vi "Arm Main copy.vi"() -> ()   [LabVIEW 2013]
doc: "This example shows how to move a motor connected to an encoder and a wheel, and then read information about the system from an encoder.\n\nThis is an example of how to use feedback (from the encoder) to create an open loop system. If some control method was used, for example using PID, a closed loop system could be created."
uses:
  Robot Global Data.vi
  Controller 2.vi
panel:
  in  "Movement Incr. Travel":dbl=1.0
  in  "Upper Limit":dbl=0.3 format="%#_13g"
  in  "Lower Limit":dbl=-0.5 format="%#_13g"
  in  "Movement Incr. Picking Up":dbl=1.0
  out "Arm Angle":dbl(graph)=148.31089863414002
  in  "Pickup Position":dbl=90.0
  out "Motor Output":dbl(graph)=0.11689101365859983
  in  "Arm Gain":dbl=0.02
  in  "Multiplier":dbl=1.0
  out "Desired Angle":dbl=160.0
  in  "Travel Position":dbl=160.0
  out "Arm Angle (deg)":dbl(knob)=148.31089863414002 scale=0.0..360.0 scale format="%#_3g"
  # "Output information."
  # "20 msec is drive\nsttion time"
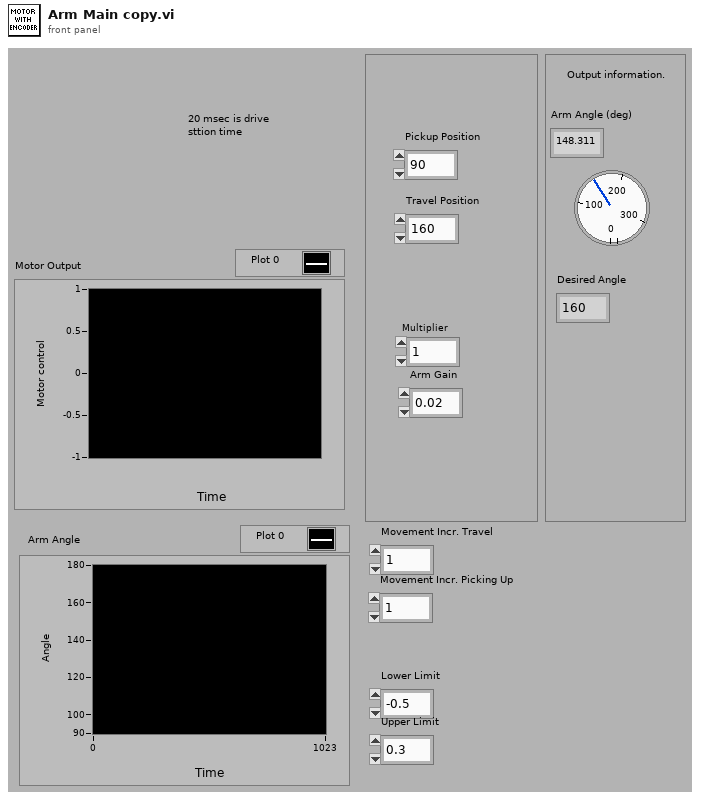
[diagram p1: front panel]
types:
  T1 = cluster{"LS X":dbl, "LS Y":dbl, "Triggers":dbl, "RS X":dbl, "RS Y":dbl}
  T2 = cluster{"A":bool, "B":bool, "X":bool, "Y":bool, "LB":bool, "RB":bool, "Back":bool, "Start":bool, "LS":bool, "RS":bool}
  T3 = typedef "WPI_EncoderDevRef.ctl" = cluster{"DevStatus":errorcluster, "EncoderIndex":T4, "CounterIndex":T5, "DistancePerCount":dbl, "Decoding Type":T6}
  T4 = typedef "FPGA_EncoderIdx.ctl" = enum8{"Enc 0", "Enc 1", "Enc 2", "Enc 3", "Invalid"}
  T5 = typedef "FPGA_CounterCtrSystemIndex.ctl" = enum8{"Ctr 0", "Ctr 1", "Ctr 2", "Ctr 3", "Ctr 4", "Ctr 5", "Ctr 6", "Ctr 7", "Invalid"}
  T6 = typedef "WPI_EncoderType.ctl" = enum16{"1x", "2x", "4x"}
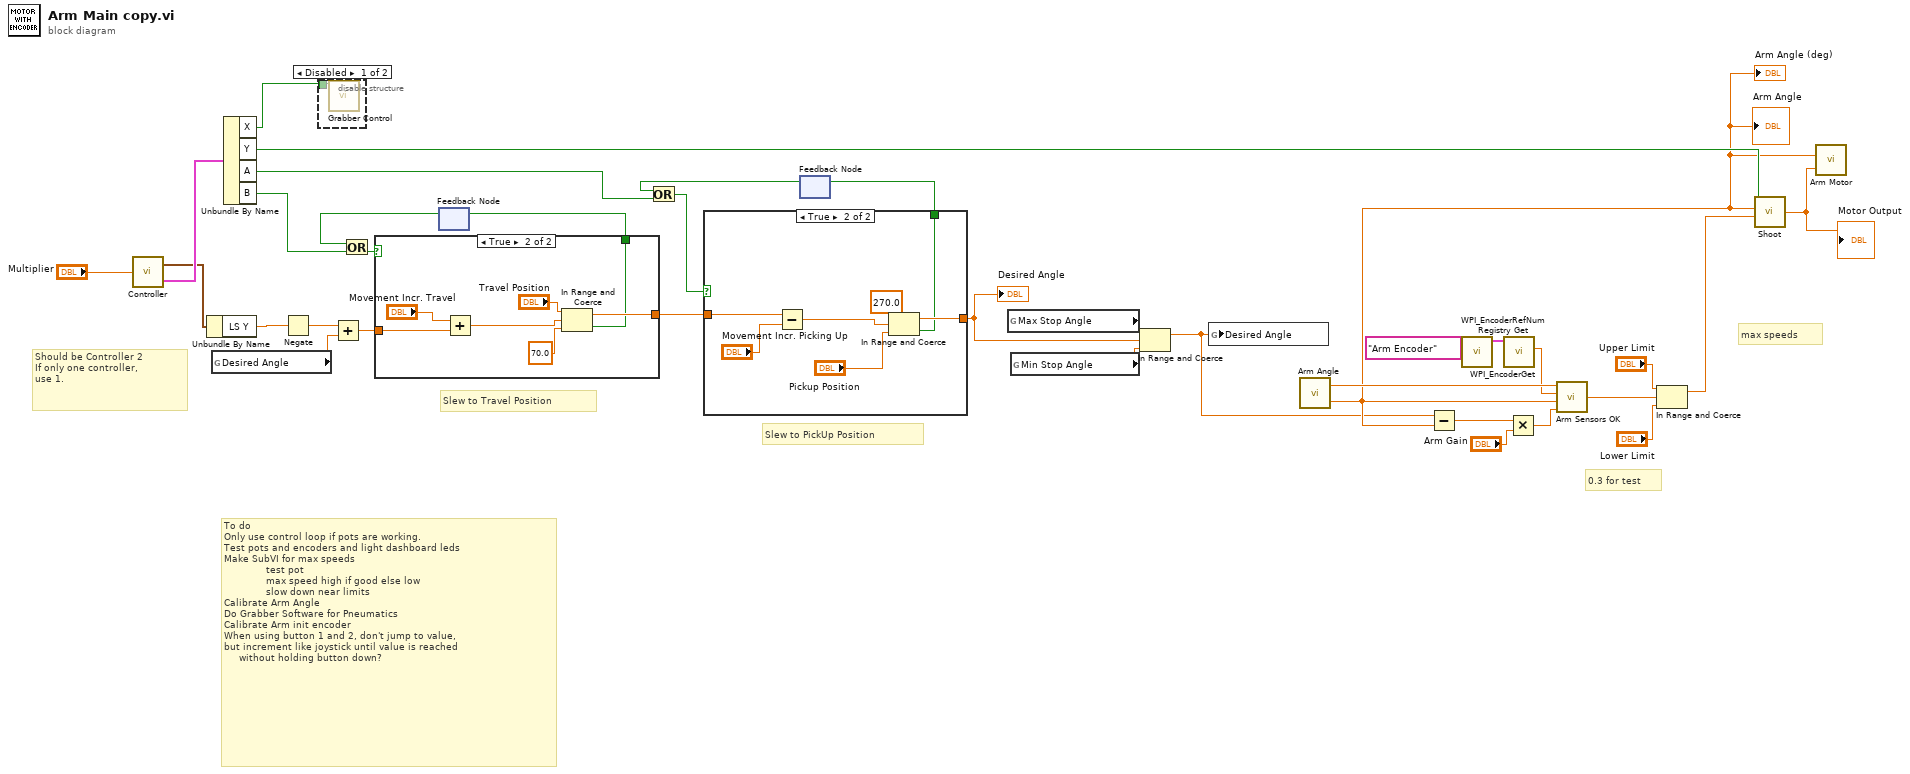
[diagram p0: block diagram]
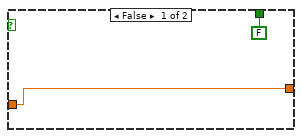
[diagram p3: hidden frame]
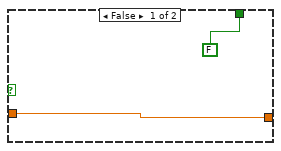
[diagram p4: hidden frame]
diagram:
  # "Slew to PickUp Position"
  # "Slew to Travel Position"
  # "Should be Controller 2\nIf only one controller, \nuse 1."
  # "0.3 for test"
  # "max speeds"
  # "To do\nOnly use control loop if pots are working. \nTest pots and encoders and light dashboard leds\nMake SubVI for max speeds \n              test pot\n              max speed high if good else low\n              slow down near limits\nCalibrate Arm Angle\nDo Grabber Software for Pneumatics\nCalibrate Arm init encoder\nWhen using button 1 and 2, don't jump to value,                                      but increment like joystick until value is reached\n     without holding button down?"
  n1 = call-poly "Controller.vi"("Joystick Multiplier"="Multiplier") -> ("Axes"=w18:T1, "Buttons"=w19:T2)
  n2 = Unbundle By Name(w18) -> ("LS Y"=w16:dbl)
  n3 = global read "Robot Global Data.vi" "Desired Angle"() -> (w9:dbl)
  n4 = Unbundle By Name(w19) -> ("X"=w14:bool, "Y"=w13:bool, "A"=w3:bool, "B"=w15:bool)
  n5 = Negate(x=w16) -> (-x=w32:dbl)
  n6 = disable-structure shown="Disabled" {
    disable-tunnel: w14 -> [w36 _]
    frame Disabled {
      n7 = call "Grabber Control.vi"("Open"=w36) -> ()  [unwired: 2 in]
    }
    frame Enabled {
    }
  }
  n8 = Add(x=w32, y=w9) -> (x+y=w28:dbl)
  n9 = feedback #1() -> (w5:bool)  [unwired: 1 in]
  n10 = Or(x=w5, y=w15) -> (x .or. y?=w7:bool)
  n11 = case shown="True" w7 {
    tunnel: [w38 w42] -> w27
    tunnel: w28 -> [w38 w45]
    tunnel: [FALSE w39] -> w6
    frame False {
    }
    frame True {
      n12 = Add(x="Movement Incr. Travel", y=w45) -> (x+y=w43:dbl)
      n13 = In Range and Coerce(upper limit="Travel Position", x=w43, lower limit=70.0) -> (coerced(x)=w42:dbl, In Range?=w39:bool)
    }
  }
  n14 = feedback-in #1(w6) -> ()
  n15 = feedback #2() -> (w1:bool)  [unwired: 1 in]
  n16 = Or(x=w1, y=w3) -> (x .or. y?=w4:bool)
  n17 = case shown="True" w4 {
    tunnel: [w47 w50] -> w26
    tunnel: w27 -> [w47 w54]
    tunnel: [FALSE w48] -> w2
    frame False {
    }
    frame True {
      n18 = Subtract(x=w54, y="Movement Incr. Picking Up") -> (x-y=w52:dbl)
      n19 = In Range and Coerce(upper limit=270.0, x=w52, lower limit="Pickup Position") -> (coerced(x)=w50:dbl, In Range?=w48:bool)
    }
  }
  "Desired Angle" <- w26
  n20 = feedback-in #2(w2) -> ()
  n21 = global read "Robot Global Data.vi" "Max Stop Angle"() -> (w12:dbl)
  n22 = global read "Robot Global Data.vi" "Min Stop Angle"() -> (w11:dbl)
  n23 = In Range and Coerce(upper limit=w12, x=w26, lower limit=w11) -> (coerced(x)=w8:dbl)  [unwired: 1 out]
  n24 = global write "Robot Global Data.vi" "Desired Angle"(w8) -> ()
  n25 = call "Arm Angle.vi"() -> ("Angle"=w10:dbl, "Voltage"=w23:dbl)  [unwired: 2 in]
  "Arm Angle (deg)" <- w10
  "Arm Angle" <- w10
  n26 = Subtract(x=w8, y=w10) -> (x-y=w35:dbl)
  n27 = call <vilib>:"WPI_EncoderRefNum Registry Get.vi"("refnum name"="Arm Encoder") -> ("EncoderDevRef"=w21:T3)  [unwired: 9 in, 1 out]
  n28 = call <vilib>:"WPI_EncoderGet.vi"("EncoderDevRef"=w21) -> ("Distance"=w22:dbl)  [unwired: 5 in, 5 out]
  n29 = Multiply(x=w35, y="Arm Gain") -> (x*y=w24:dbl)
  n30 = call "Arm Sensors OK.vi"("Motor In"=w24, "Pot Angle"=w10, "Encoder Angle"=w22, "Pot Voltage"=w23) -> ("Motor Out"=w25:dbl)
  n31 = In Range and Coerce(upper limit="Upper Limit", x=w25, lower limit="Lower Limit") -> (coerced(x)=w33:dbl)  [unwired: 1 out]
  n32 = call "Shoot.vi"("Shoot"=w13, "Current Angle"=w10, "Current Motor SetPoint"=w33) -> ("New Motor Setpoint"=w31:dbl)  [unwired: 2 in]
  "Motor Output" <- w31
  n33 = call "Arm Motor.vi"("Motor input"=w31, "Current angle (deg)"=w10) -> ()  [unwired: 1 in]
